vi "sevensegment(SubVI).vi"(11 "Numeric":i32) -> ()   [LabVIEW 2017]
uses:
  <vilib>/myRIO/Common/Instrument Driver Framework/myRIO v1.0/DIO/typedefs/DIO Channels Enum.ctl
  <vilib>/myRIO/Common/Instrument Driver Framework/myRIO v1.0/DIO/typedefs/DIO Channels List.ctl
  <vilib>/myRIO/Common/Instrument Driver Framework/Utilities/typedefs/Generic FPGA Reference.ctl
  <vilib>/myRIO/Common/Instrument Driver Framework/Utilities/typedefs/myRIO v1.0 Reference.ctl
  <vilib>/myRIO/Common/Instrument Driver Framework/Utilities/typedefs/Hardware Version Enum.ctl
  <vilib>/myRIO/Common/Instrument Driver Framework/Utilities/typedefs/myRIO Generic Hardware Reference.ctl
  <vilib>/myRIO/Instrument Drivers/Onboard IO/DIO/typedefs/DIO Reference.ctl
  <vilib>/myRIO/Instrument Drivers/Onboard IO/DIO/DIO.lvlib
  <vilib>/myRIO/Instrument Drivers/Onboard IO/DIO/vis/Write.vi
  <vilib>/myRIO/Instrument Drivers/Onboard IO/DIO/vis/myRIO DIO Open.xnode
  <vilib>/myRIO/Common/Instrument Driver Framework/Utilities/vis/Is FPGA Ref Available.vi
  <vilib>/myRIO/Express VI/Onboard IO/DO/DO Express VI.xnode
  <vilib>/myRIO/Common/Instrument Driver Framework/myRIO v1.0/DIO/vis/myRIO v1.1 Open DIO.vi
  <vilib>/userdefined/High Color/nirio_resource_hc.ctl
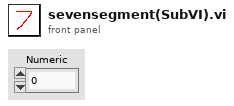
[diagram p1: front panel]
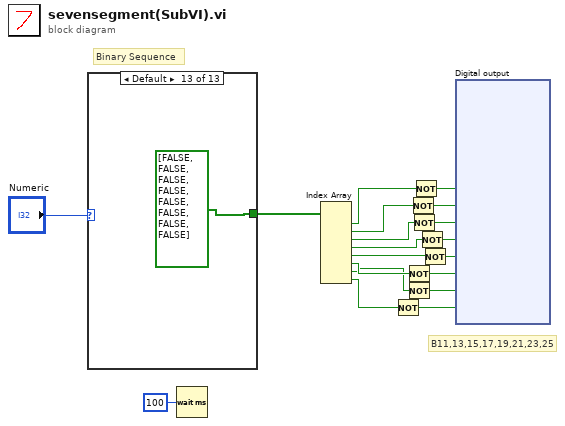
[diagram p0: block diagram]
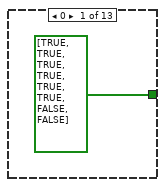
[diagram p2: hidden frame]
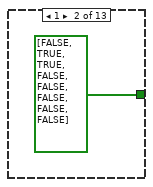
[diagram p3: hidden frame]
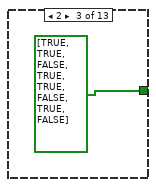
[diagram p4: hidden frame]
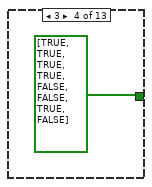
[diagram p5: hidden frame]
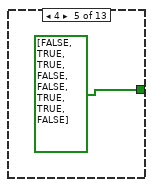
[diagram p6: hidden frame]
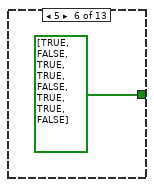
[diagram p7: hidden frame]
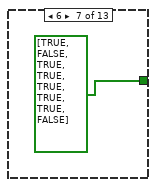
[diagram p8: hidden frame]
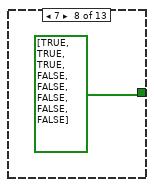
[diagram p9: hidden frame]
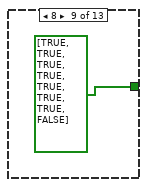
[diagram p10: hidden frame]
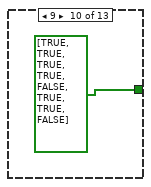
[diagram p11: hidden frame]
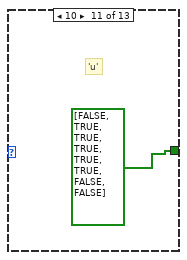
[diagram p12: hidden frame]
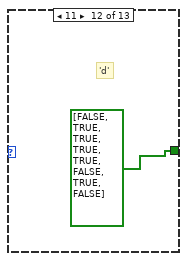
[diagram p13: hidden frame]
diagram:
  # "B11,13,15,17,19,21,23,25"
  # "Binary Sequence"
  n1 = case shown="Default" "Numeric" {
    tunnel: [bool[] [TRUE, TRUE, TRUE, TRUE, TRUE, TRUE, FALSE, FALSE] bool[] [FALSE, TRUE, TRUE, FALSE, FALSE, FALSE, FALSE, FALSE] bool[] [TRUE, TRUE, FALSE, TRUE, TRUE, FALSE, TRUE, FALSE] bool[] [TRUE, TRUE, TRUE, TRUE, FALSE, FALSE, TRUE, FALSE] bool[] [FALSE, TRUE, TRUE, FALSE, FALSE, TRUE, TRUE, FALSE] bool[] [TRUE, FALSE, TRUE, TRUE, FALSE, TRUE, TRUE, FALSE] bool[] [TRUE, FALSE, TRUE, TRUE, TRUE, TRUE, TRUE, FALSE] bool[] [TRUE, TRUE, TRUE, FALSE, FALSE, FALSE, FALSE, FALSE] bool[] [TRUE, TRUE, TRUE, TRUE, TRUE, TRUE, TRUE, FALSE] bool[] [TRUE, TRUE, TRUE, TRUE, FALSE, TRUE, TRUE, FALSE] bool[] [FALSE, TRUE, TRUE, TRUE, TRUE, TRUE, FALSE, FALSE] bool[] [FALSE, TRUE, TRUE, TRUE, TRUE, FALSE, TRUE, FALSE] bool[] [FALSE, FALSE, FALSE, FALSE, FALSE, FALSE, FALSE, FALSE]] -> w18
    frame 0 {
    }
    frame 1 {
    }
    frame 2 {
    }
    frame 3 {
    }
    frame 4 {
    }
    frame 5 {
    }
    frame 6 {
    }
    frame 7 {
    }
    frame 8 {
    }
    frame 9 {
    }
    frame 10 {
      # "'u'"
    }
    frame 11 {
      # "'d'"
    }
    frame Default {
    }
  }
  n2 = Wait (ms)(milliseconds to wait=u32 100) -> ()  [unwired: 1 out]
  n3 = Index Array(array=w18) -> (element #1=w8:bool, element #2=w7:bool, element #3=w6:bool, element #4=w5:bool, element #5=w4:bool, element #6=w3:bool, element #7=w2:bool, element #8=w1:bool)  [unwired: 8 in]
  n4 = Not(x=w1) -> (.not. x?=w9:bool)
  n5 = Not(x=w3) -> (.not. x?=w11:bool)
  n6 = Not(x=w2) -> (.not. x?=w10:bool)
  n7 = Not(x=w7) -> (.not. x?=w15:bool)
  n8 = Not(x=w6) -> (.not. x?=w14:bool)
  n9 = Not(x=w8) -> (.not. x?=w16:bool)
  n10 = Not(x=w5) -> (.not. x?=w13:bool)
  n11 = Not(x=w4) -> (.not. x?=w12:bool)
  n12 = xnode "Digital output"("B/DIO0 (Pin 11)"=w16, "B/DIO1 (Pin 13)"=w15, "B/DIO2 (Pin 15)"=w14, "B/DIO3 (Pin 17)"=w13, "B/DIO4 (Pin 19)"=w12, "B/DIO5 (Pin 21)"=w11, "B/DIO6 (Pin 23)"=w10, "B/DIO7 (Pin 25)"=w9) -> ()  [unwired: 1 in, 1 out]
